vi "Initialize.vi"(8 "Debug Alias":string, 9 "Open Actor Core front panel? (F)":bool, 10 "Auto-stop? (T)":bool=TRUE, 11 "Nested Actor":refnum<class "Actor.lvclass">) -> (3 "Launch Nested Actor Msg":refnum<class "Launch Nested Actor Msg.lvclass">)   [LabVIEW 2020, in "Actor Framework.lvlib" / "Launch Nested Actor Msg.lvclass"]
doc: "This VI initializes the fields of an instance of Launch Nested Actor Msg.lvclass."
uses:
  Launch Nested Actor Msg.lvclass
  Actor/Actor.lvclass
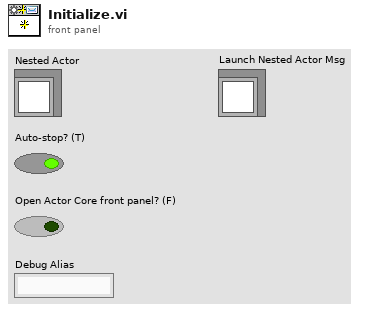
[diagram p1: front panel]
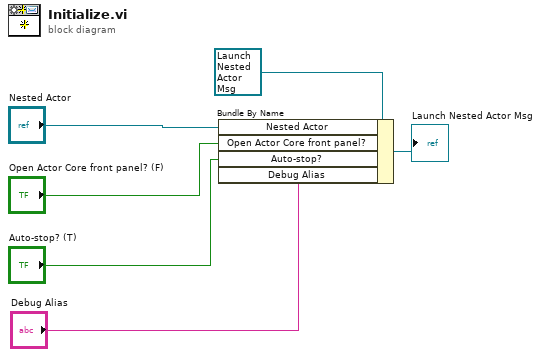
[diagram p0: block diagram]
diagram:
  n1 = Bundle By Name(cluster=refnum<class "Launch Nested Actor Msg.lvclass"> refnum ("Launch Nested Actor Msg"), "Nested Actor"="Nested Actor", "Open Actor Core front panel?"="Open Actor Core front panel? (F)", "Auto-stop?"="Auto-stop? (T)", "Debug Alias"="Debug Alias") -> (→"Launch Nested Actor Msg":refnum<class "Launch Nested Actor Msg.lvclass">)
